vi "Set Refs.vi"(4 "Display Direction in":refnum<vi>, 5 "Display Action Info in":refnum<vi>, 6 "VI ref in":refnum<vi>, 7 "Game Board ref in":refnum<vi>, 8 "Display info in":refnum<vi>, 9 "Score right in":refnum<vi>, 10 "Score left in":refnum<vi>) -> (3 "Game Board out":refnum<class "Game Board.lvclass">)   [LabVIEW 2021, in "Game Board.lvclass"]
doc: "MIT Licence\nCopyright (c) 2024 David Grollier"
uses:
  Game Board.lvclass
  Game Board.lvclass/Game Board.ctl
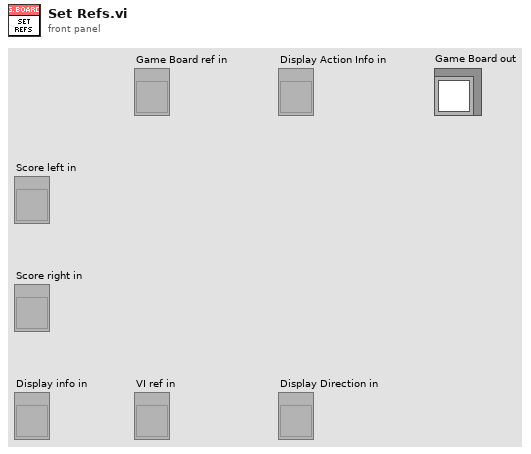
[diagram p1: front panel]
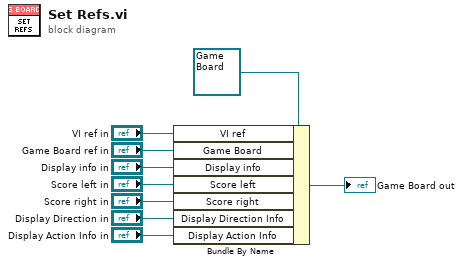
[diagram p0: block diagram]
diagram:
  n1 = Bundle By Name(cluster=refnum<class "Game Board.lvclass"> refnum ("Game Board out"), "VI ref"="VI ref in", "Game Board"="Game Board ref in", "Display info"="Display info in", "Score left"="Score left in", "Score right"="Score right in", "Display Direction Info"="Display Direction in", "Display Action Info"="Display Action Info in") -> (→"Game Board out":refnum<class "Game Board.lvclass">)
